vi "PLL Lock.vi"(8 "error in (no error)":errorcluster, 10 "PLL lock  (T: Enable)":bool=TRUE, 11 "VISA resource name":refnum<visa-resource-name>) -> (0 "error out":errorcluster, 3 "VISA resource name out":refnum<visa-resource-name>)   [LabVIEW 2013, in "AWG.lvlib" / "Agilent 33XXX Series.lvlib"]
doc: "Enables or disables phase lock to 10 MHz reference input."
uses:
  Agilent 33XXX Series.lvlib
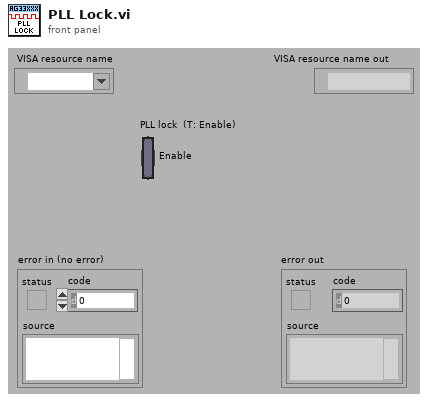
[diagram p1: front panel]
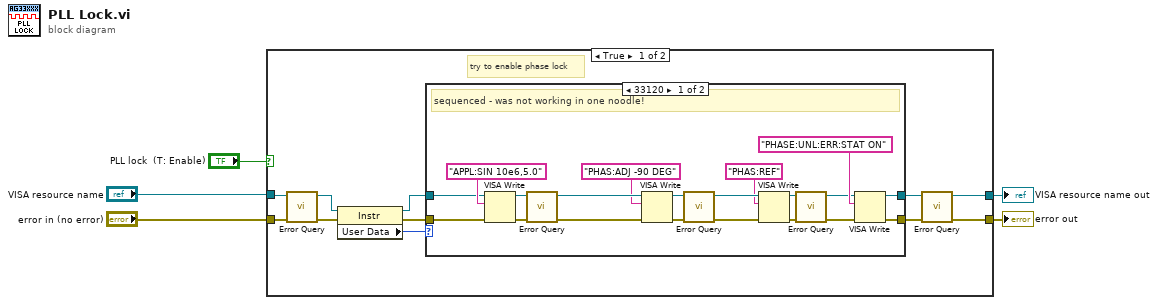
[diagram p0: block diagram]
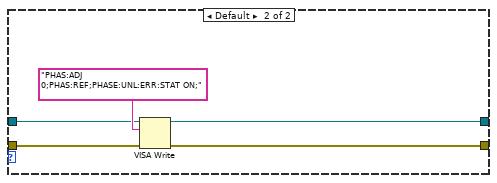
[diagram p2: hidden frame]
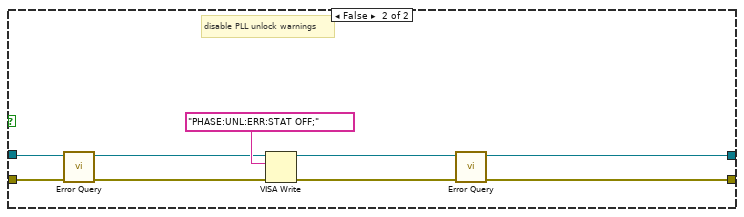
[diagram p3: hidden frame]
diagram:
  n1 = case shown="True" "PLL lock  (T: Enable)" {
    tunnel: [w14 w48] -> w4
    tunnel: [w13 w47] -> w5
    tunnel: "VISA resource name" -> [w11 w44]
    tunnel: "error in (no error)" -> [w12 w45]
    frame True {
      # "try to enable phase lock"
      n2 = call "Error Query.vi"("error in (no error)"=w12, "VISA resource name"=w11) -> ("error out"=w10:errorcluster, "VISA resource name out"=w9:refnum<visa-resource-name>)  [unwired: 6 in, 2 out]
      n3 = property class="Instr"(reference=w9, error in=w10) -> (reference out=w7:refnum<visa-resource-name>, error out=w8:errorcluster, "User Data"=w6:u32)
      n4 = case shown="33120" w6 {
        tunnel: [w20 w41] -> w16
        tunnel: [w19 w40] -> w15
        tunnel: w7 -> [w35 w38]
        tunnel: w8 -> [w34 w37]
        frame 33120 {
          # "sequenced - was not working in one noodle!"
          n5 = VISA Write(VISA resource name=w35, write buffer="APPL:SIN 10e6,5.0", error in (no error)=w34) -> (VISA resource name out=w32:refnum<visa-resource-name>, error out=w33:errorcluster)  [unwired: 1 out]
          n6 = call "Error Query.vi"("error in (no error)"=w33, "VISA resource name"=w32) -> ("error out"=w30:errorcluster, "VISA resource name out"=w31:refnum<visa-resource-name>)  [unwired: 6 in, 2 out]
          n7 = VISA Write(VISA resource name=w31, write buffer="PHAS:ADJ -90 DEG", error in (no error)=w30) -> (VISA resource name out=w25:refnum<visa-resource-name>, error out=w26:errorcluster)  [unwired: 1 out]
          n8 = call "Error Query.vi"("error in (no error)"=w26, "VISA resource name"=w25) -> ("error out"=w28:errorcluster, "VISA resource name out"=w27:refnum<visa-resource-name>)  [unwired: 6 in, 2 out]
          n9 = VISA Write(VISA resource name=w27, write buffer="PHAS:REF", error in (no error)=w28) -> (VISA resource name out=w18:refnum<visa-resource-name>, error out=w17:errorcluster)  [unwired: 1 out]
          n10 = call "Error Query.vi"("error in (no error)"=w17, "VISA resource name"=w18) -> ("error out"=w21:errorcluster, "VISA resource name out"=w22:refnum<visa-resource-name>)  [unwired: 6 in, 2 out]
          n11 = VISA Write(VISA resource name=w22, write buffer="PHASE:UNL:ERR:STAT ON", error in (no error)=w21) -> (VISA resource name out=w19:refnum<visa-resource-name>, error out=w20:errorcluster)  [unwired: 1 out]
        }
        frame Default {
          n12 = VISA Write(VISA resource name=w38, write buffer="PHAS:ADJ 0;PHAS:REF;PHASE:UNL:ERR:STAT ON;", error in (no error)=w37) -> (VISA resource name out=w40:refnum<visa-resource-name>, error out=w41:errorcluster)  [unwired: 1 out]
        }
      }
      n13 = call "Error Query.vi"("error in (no error)"=w16, "VISA resource name"=w15) -> ("error out"=w13:errorcluster, "VISA resource name out"=w14:refnum<visa-resource-name>)  [unwired: 6 in, 2 out]
    }
    frame False {
      # "disable PLL unlock warnings"
      n14 = call "Error Query.vi"("error in (no error)"=w45, "VISA resource name"=w44) -> ("error out"=w42:errorcluster, "VISA resource name out"=w43:refnum<visa-resource-name>)  [unwired: 6 in, 2 out]
      n15 = VISA Write(VISA resource name=w43, write buffer="PHASE:UNL:ERR:STAT OFF;", error in (no error)=w42) -> (VISA resource name out=w49:refnum<visa-resource-name>, error out=w50:errorcluster)  [unwired: 1 out]
      n16 = call "Error Query.vi"("error in (no error)"=w50, "VISA resource name"=w49) -> ("error out"=w47:errorcluster, "VISA resource name out"=w48:refnum<visa-resource-name>)  [unwired: 6 in, 2 out]
    }
  }
  "error out" <- w5
  "VISA resource name out" <- w4
